vi "Draw_Shape_Ellipses.vi"(6 "Color":u32(colorbox)=16711680, 8 "error in":errorcluster, 10 "Ellipse Descriptor":T1, 11 "Image":T2) -> (0 "error out":errorcluster, 3 "Image Out":T2)   [LabVIEW 2019]
uses:
  <vilib>/vision/Image Controls.llb/IMAQ Image.ctl
panel:
  in  "Group":string
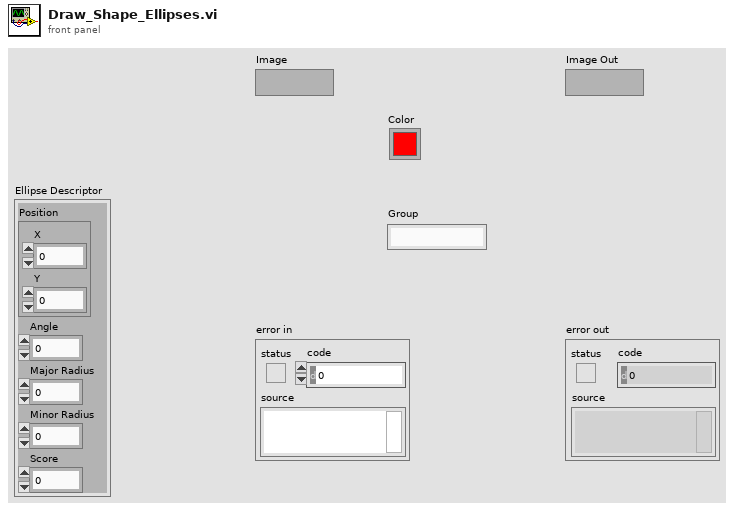
[diagram p1: front panel]
types:
  T1 = cluster{"Position":cluster{"X":sgl, "Y":sgl}, "Angle":dbl, "Major Radius":dbl, "Minor Radius":dbl, "Score":dbl}
  T2 = typedef "IMAQ Image.ctl" = refnum<image>
  T3 = cluster{dbl, dbl, "Major Radius":dbl, "Minor Radius":dbl}
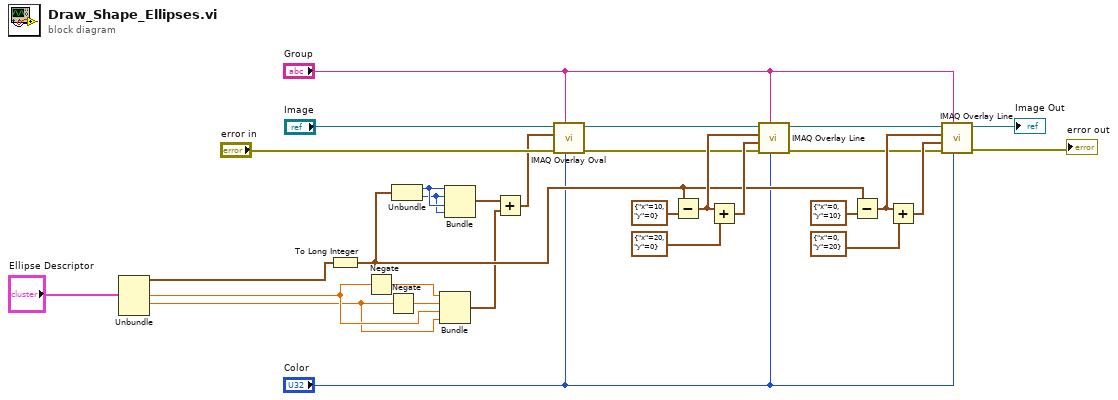
[diagram p0: block diagram]
diagram:
  n1 = Unbundle("Ellipse Descriptor") -> ("Position"=w10:cluster{"X":sgl, "Y":sgl}, "Major Radius"=w9:dbl, "Minor Radius"=w8:dbl)  [unwired: 2 out]
  n2 = To Long Integer(number=w10) -> (32bit integer=w15:cluster{"X":i32, "Y":i32})
  n3 = Negate(x=w9) -> (-x=w13:dbl)
  n4 = Negate(x=w8) -> (-x=w12:dbl)
  n5 = Unbundle(w15) -> ("X"=w28:i32, "Y"=w27:i32)
  n6 = Bundle(w13, w12, "Major Radius"=w9, "Minor Radius"=w8) -> (w11:T3)  [unwired: 1 in]
  n7 = Bundle("X"=w28, "Y"=w27, "X"=w28, "Y"=w27) -> (w26:cluster{"X":i32, "Y":i32, "X":i32, "Y":i32})  [unwired: 1 out]
  n8 = Add(x=w26, y=w11) -> (x+y=w5:cluster{dbl, dbl, dbl, dbl})
  n9 = call "IMAQ Overlay Oval"("Color"="Color", "Group"="Group", "error in (no error)"="error in", "Bounding Rectangle"=w5, "Image"="Image") -> ("error out"=w2:errorcluster, "Image Out"=w3:T2)  [unwired: 5 in]
  n10 = Subtract(x=w15, y=cluster{"x":i32, "y":i32} {"x"=10, "y"=0}) -> (x-y=w24:cluster{i32, i32})
  n11 = Add(x=w24, y=cluster{"x":i32, "y":i32} {"x"=20, "y"=0}) -> (x+y=w22:cluster{i32, i32})
  n12 = call "IMAQ Overlay Line"("Color"="Color", "Group"="Group", "error in (no error)"=w2, "End Point"=w22, "Start Point"=w24, "Image"=w3) -> ("error out"=w16:errorcluster, "Image Out"=w17:T2)  [unwired: 4 out]
  n13 = Subtract(x=w15, y=cluster{"x":i32, "y":i32} {"x"=0, "y"=10}) -> (x-y=w20:cluster{i32, i32})
  n14 = Add(x=w20, y=cluster{"x":i32, "y":i32} {"x"=0, "y"=20}) -> (x+y=w21:cluster{i32, i32})
  n15 = call "IMAQ Overlay Line"("Color"="Color", "Group"="Group", "error in (no error)"=w16, "End Point"=w21, "Start Point"=w20, "Image"=w17) -> ("error out"=→"error out":errorcluster, "Image Out"=→"Image Out":T2)  [unwired: 4 out]
